vi "pH电极校准.vi"() -> ()   [LabVIEW 2016, in "国弘多参数.lvlib"]
panel:
  out "当前检测值":dbl
  out "提示":string
  in  "第二点通过校正":bool
  in  "第一点通过校正":bool
  in  "第二点校正":bool
  in  "第一点校正":bool
  out "标液2":dbl
  out "标液1":dbl
  out "当前信号值":dbl
  out "偏移值补偿":dbl
  out "电极斜率":dbl
  out "电极零点":dbl
  # "酸碱度电极设定"
  # "mV"
  # "pH"
  # "%"
  # "mV"
  # "电极校正"
  # "标准液值:"
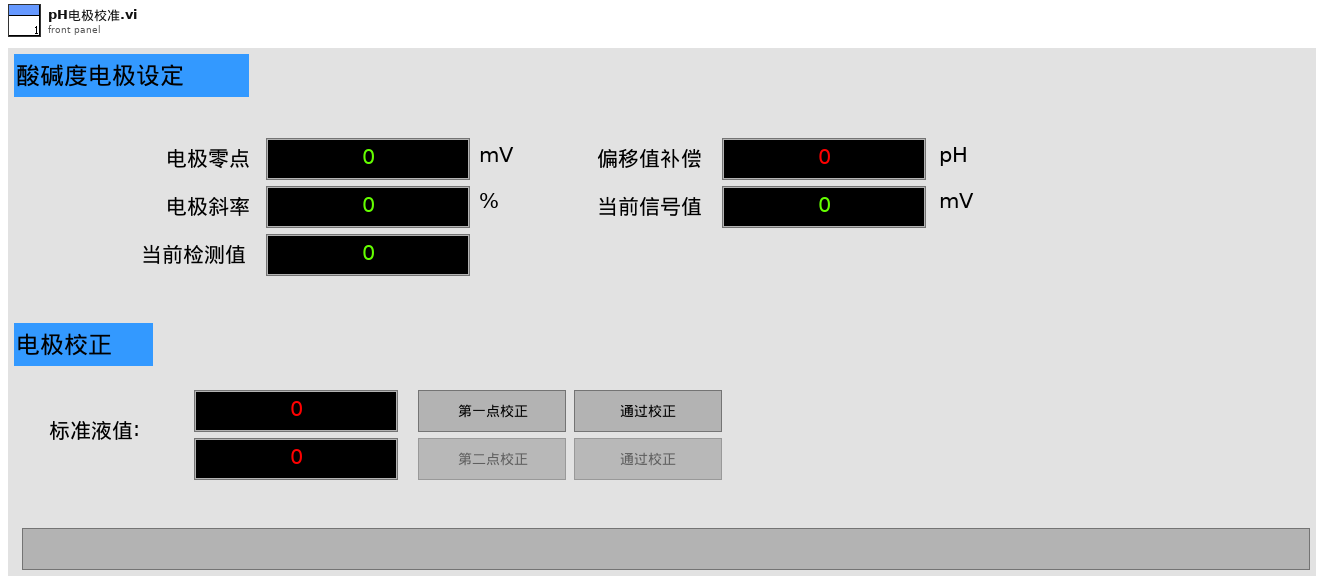
[diagram p1: front panel]
types:
  T1 = enum8{"Enabled", "Disabled", "Disabled and Grayed Out"}
  T2 = enum16{"待机", "第一点校准", "第一点校准通过", "第二点校准", "第二点校准通过", "等待数据稳定"}
  T3 = cluster{"电极状态标志":u16, "电极型号标志":u16, "酸碱度测量值":sgl, "温度测量值":sgl, "酸碱度信号值":sgl, "温度信号值":sgl, "酸碱度偏移修正值":sgl, "温度偏移修正值":sgl, "手动温度补偿值":sgl, "酸碱度电极零点":sgl, "酸碱度电极斜率":sgl, "第1点标准值记录":sgl, "第1点信号值记录":sgl, "第1点温度值记录":sgl, "第2点标准值记录":sgl, "第2点信号值记录":sgl, "第2点温度值记录":sgl, "命令滤波设定":u16, "温度模式":enum16{"ATC", "MTC"}, "生产批次":u16, "电极序号":u16, "串口地址":u16, "串口波特率":enum16{"9600", "19200", "115200"}, "串口校验位":enum16{"NONE", "ODD", "EVEN"}, "串口停止位":enum16{"1bit", "2bit"}, "第一点标准值":sgl, "第二点标准值":sgl}
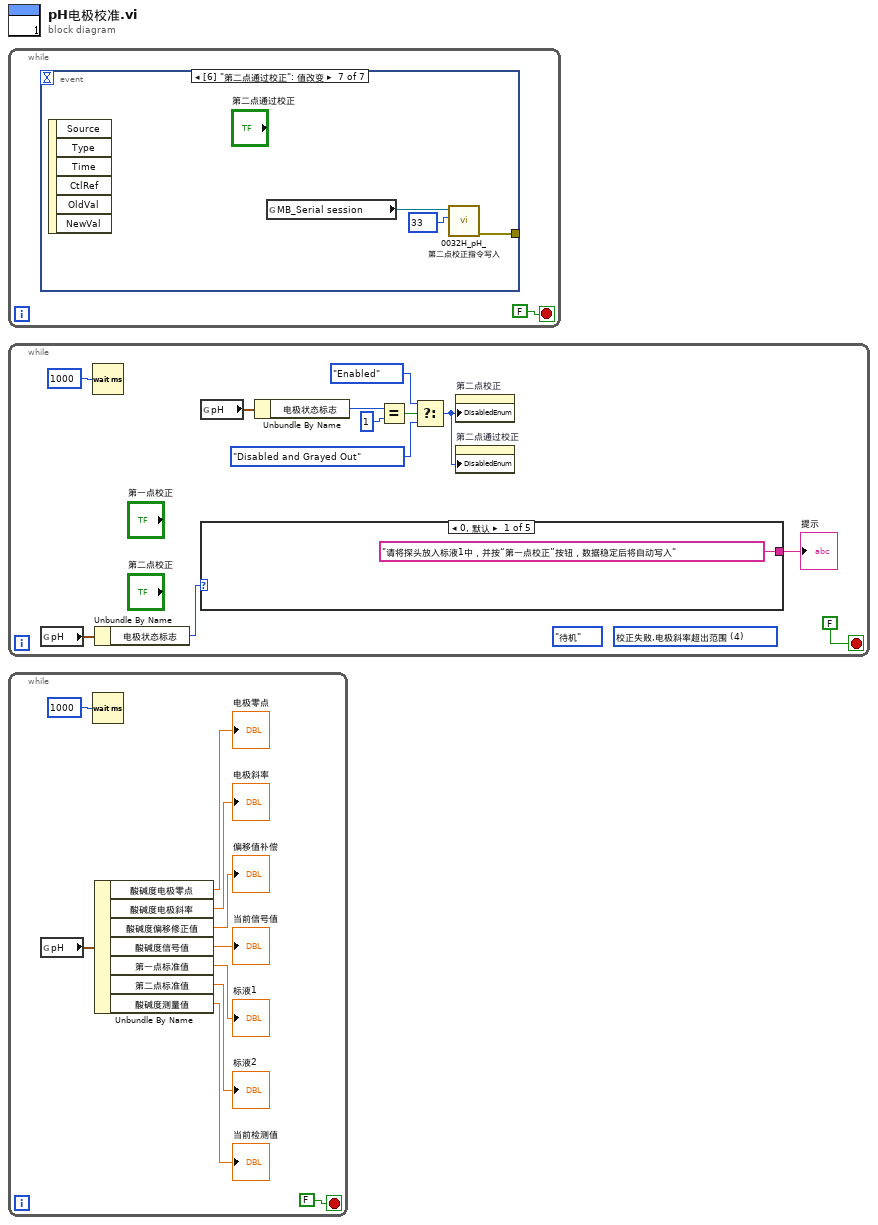
[diagram p0: block diagram]
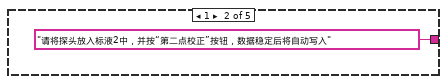
[diagram p2: hidden frame]
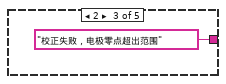
[diagram p3: hidden frame]
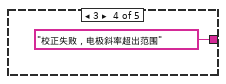
[diagram p4: hidden frame]
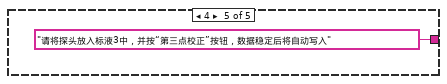
[diagram p5: hidden frame]
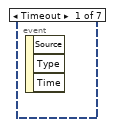
[diagram p6: hidden frame]
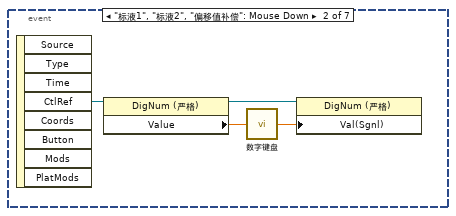
[diagram p7: hidden frame]
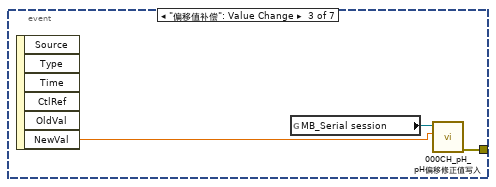
[diagram p8: hidden frame]
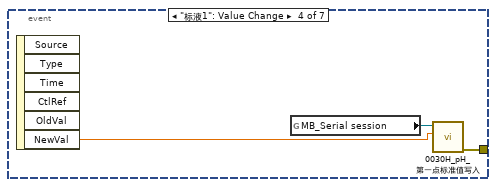
[diagram p9: hidden frame]
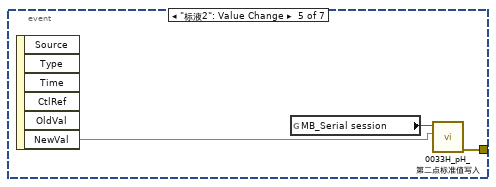
[diagram p10: hidden frame]
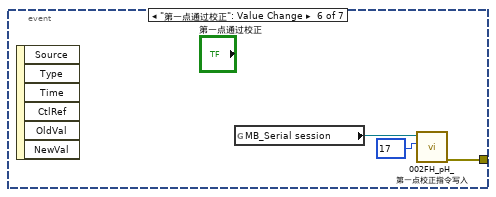
[diagram p11: hidden frame]
diagram:
  n1 = while {
    stop <- FALSE stop-if-true
    n2 = event shown="[6] \"第二点通过校正\": 值改变" {
      selector: _ -> [_ _ _ _ _ _ _]
      dyn-events: _ -> [_ _ _ _ _ _ _]
      timeout: _ -> [_ _ _ _ _ _ _]
      tunnel: [_ _ w6 w9 w12 w15 w18] -> _
      event Timeout {
        n3 = event-data() -> ()  [unwired: 1 in, 3 out]
      }
      event "标液1", "标液2", "偏移值补偿": Mouse Down {
        n4 = event-data() -> ("CtlRef"=w5:refnum<vi>)  [unwired: 1 in, 7 out]
        n5 = property class="DigNum (严格)"(reference=w5) -> (reference out=w2:refnum<vi>, "Value"=w3:dbl)  [unwired: 1 in, 1 out]
        n6 = call "数字键盘.vi"("OldNumber"=w3) -> ("NewNumber"=w4:sgl)
        n7 = property class="DigNum (严格)"(reference=w2, "Val(Sgnl)"=w4) -> ()  [unwired: 1 in, 2 out]
      }
      event "偏移值补偿": Value Change {
        n8 = event-data() -> ("NewVal"=w8:dbl)  [unwired: 1 in, 5 out]
        n9 = global read "过程全局变量.vi" "MB_Serial session"() -> (w7:refnum<class "MB_Master_Serial.lvclass">)
        n10 = call "000CH_pH_pH偏移修正值写入.vi"("数值"=w8, "MB_Serial session in"=w7) -> ("error out"=w6:errorcluster)  [unwired: 8 in, 1 out]
      }
      event "标液1": Value Change {
        n11 = event-data() -> ("NewVal"=w10:dbl)  [unwired: 1 in, 5 out]
        n12 = global read "过程全局变量.vi" "MB_Serial session"() -> (w11:refnum<class "MB_Master_Serial.lvclass">)
        n13 = call "0030H_pH_第一点标准值写入.vi"("数值"=w10, "MB_Serial session in"=w11) -> ("error out"=w9:errorcluster)  [unwired: 8 in, 1 out]
      }
      event "标液2": Value Change {
        n14 = event-data() -> ("NewVal"=w13:dbl)  [unwired: 1 in, 5 out]
        n15 = global read "过程全局变量.vi" "MB_Serial session"() -> (w14:refnum<class "MB_Master_Serial.lvclass">)
        n16 = call "0033H_pH_第二点标准值写入.vi"("数值"=w13, "MB_Serial session in"=w14) -> ("error out"=w12:errorcluster)  [unwired: 8 in, 1 out]
      }
      event "第一点通过校正": Value Change {
        n17 = event-data() -> ()  [unwired: 1 in, 6 out]
        n18 = global read "过程全局变量.vi" "MB_Serial session"() -> (w17:refnum<class "MB_Master_Serial.lvclass">)
        n19 = call "002FH_pH_第一点校正指令写入.vi"("数值"=u16 17, "MB_Serial session in"=w17) -> ("error out"=w15:errorcluster)  [unwired: 8 in, 1 out]
      }
      event "第二点通过校正": Value Change {
        n20 = event-data() -> ()  [unwired: 1 in, 6 out]
        n21 = global read "过程全局变量.vi" "MB_Serial session"() -> (w20:refnum<class "MB_Master_Serial.lvclass">)
        n22 = call "0032H_pH_第二点校正指令写入.vi"("数值"=u16 33, "MB_Serial session in"=w20) -> ("error out"=w18:errorcluster)  [unwired: 8 in, 1 out]
      }
    }
  }
  n23 = while {
    stop <- FALSE stop-if-true
    (unwired) u16 4 items=["OK", "第一点校正通过", "第二点校正通过", "校正失败,电极零点超出范围", "校正失败,电极斜率超出范围", "第三点校正通过"] ("电极状态标志")
    (unwired) T2."待机" ("枚举")
    n24 = global read "过程全局变量.vi" "pH"() -> (w23:T3)
    n25 = Wait (ms)(milliseconds to wait=u32 1000 ("等待时间（毫秒）")) -> ()  [unwired: 1 out]
    n26 = Unbundle By Name(w23) -> ("电极状态标志"=w22:u16)
    n27 = global read "过程全局变量.vi" "pH"() -> (w30:T3)
    n28 = case shown="0, 默认" w22 {
      tunnel: ["请将探头放入标液1中，并按“第一点校正”按钮，数据稳定后将自动写入" ("提示") "请将探头放入标液2中，并按“第二点校正”按钮，数据稳定后将自动写入" ("提示") "校正失败，电极零点超出范围" ("提示") "校正失败，电极斜率超出范围" ("提示") "请将探头放入标液3中，并按“第三点校正”按钮，数据稳定后将自动写入" ("提示")] -> w21
      frame 0, Default {
      }
      frame 1 {
      }
      frame 2 {
      }
      frame 3 {
      }
      frame 4 {
      }
    }
    "提示" <- w21
    n29 = Unbundle By Name(w30) -> ("电极状态标志"=w29:u16)
    n30 = Equal?(x=w29, y=u16 1) -> (x = y?=w24:bool)
    n31 = Select(t=T1."Enabled" ("禁用"), s=w24, f=T1."Disabled and Grayed Out" ("禁用")) -> (s? t:f=w25:T1)
    n32 = property on="第二点校正" class="Bool"("DisabledEnum"=w25) -> ()  [unwired: 2 in, 2 out]
    n33 = property on="第二点通过校正" class="Bool"("DisabledEnum"=w25) -> ()  [unwired: 2 in, 2 out]
  }
  n34 = while {
    stop <- FALSE stop-if-true
    n35 = global read "过程全局变量.vi" "pH"() -> (w45:T3)
    n36 = Wait (ms)(milliseconds to wait=u32 1000 ("等待时间（毫秒）")) -> ()  [unwired: 1 out]
    n37 = Unbundle By Name(w45) -> ("酸碱度电极零点"=→"电极零点":sgl, "酸碱度电极斜率"=→"电极斜率":sgl, "酸碱度偏移修正值"=→"偏移值补偿":sgl, "酸碱度信号值"=→"当前信号值":sgl, "第一点标准值"=→"标液1":sgl, "第二点标准值"=→"标液2":sgl, "酸碱度测量值"=→"当前检测值":sgl)
  }
